vi "dfd_FXP Casting (vector).vi"(5 "quantization settings":T4={"source"=6, "wl"=1, "iwl"=1, "overflow mode"=enum."Saturation", "rounding mode"=enum."Nearest", "signed?"=TRUE} {"source" items=["Coef a/k"=0, "Coef b/v"=7, "Input"=1, "Output"=2, "Multiplicand"=3, "Product"=4, "Sum"=5, "Delay"=6, "Gain"=8]}, 6 "filtering statistics in":T3(array[cluster]) {"statistics information"."min value" format="%.2f"; "statistics information"."max value" format="%.2f"; "Quantizer Source" items=["Coefficients a/k"=0, "Coefficients b/v"=7, "Input"=1, "Output"=2, "Multiplicand"=3, "Product"=4, "Sum"=5, "Delay"=6]}, 9 "values in":dbl[](array[numeric]) format="%.2f") -> (0 "filtering statistics out":T3(array[cluster]) {"statistics information"."min value" format="%.2f"; "statistics information"."max value" format="%.2f"; "Quantizer Source" items=["Coefficients a/k"=0, "Coefficients b/v"=7, "Input"=1, "Output"=2, "Multiplicand"=3, "Product"=4, "Sum"=5, "Delay"=6]}, 2 "statistics information":T2 {"min value" format="%.2f"; "max value" format="%.2f"}, 3 "values out":dbl[](array[numeric]) format="%.2f")   [LabVIEW 2017, in "NI_DigFilter_FXP.lvlib"]
uses:
  <vilib>/addons/Digital Filter Design/NI_DigFilter_FXP.lvlib
  <vilib>/addons/Digital Filter Design/_Objects.llb/dfd_Internal Quantization Settings.ctl
  <vilib>/addons/Digital Filter Design/_Objects.llb/dfd_Internal Quantization Srcs.ctl
  <vilib>/addons/Digital Filter Design/_Objects.llb/DFD FXP Statistics Data.ctl
  <vilib>/addons/Digital Filter Design/_Objects.llb/DFD Quantization Sources.ctl
  <vilib>/addons/Digital Filter Design/FXPLib.llb/dfd_FXP Overflow (vector).vi
  <vilib>/addons/Digital Filter Design/FXPLib.llb/dfd_FXP Quantization (vector).vi
  <vilib>/addons/Digital Filter Design/NI_DigFilterLicensed.lvlib
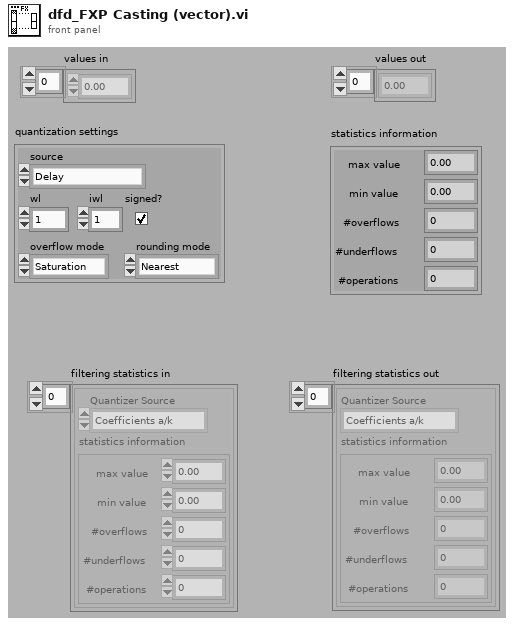
[diagram p1: front panel]
types:
  T1 = typedef "NI_DigFilterLicensed.lvlib/DFD Quantization Sources.ctl" = u16
  T2 = typedef "NI_DigFilterLicensed.lvlib/DFD FXP Statistics Data.ctl" = cluster{"max value":ext, "min value":ext, "#overflows":i32, "#underflows":i32, "#operations":i32}
  T3 = cluster{"Quantizer Source":T1, "statistics information":T2}[]
  T4 = typedef "NI_DigFilterLicensed.lvlib/dfd_Internal Quantization Settings.ctl" = cluster{"source":T5, "wl":i16, "iwl":i16, "overflow mode":enum16{"Saturation", "Wrap"}, "rounding mode":enum16{"Nearest", "Truncation"}, "signed?":bool}
  T5 = typedef "NI_DigFilterLicensed.lvlib/dfd_Internal Quantization Srcs.ctl" = u16
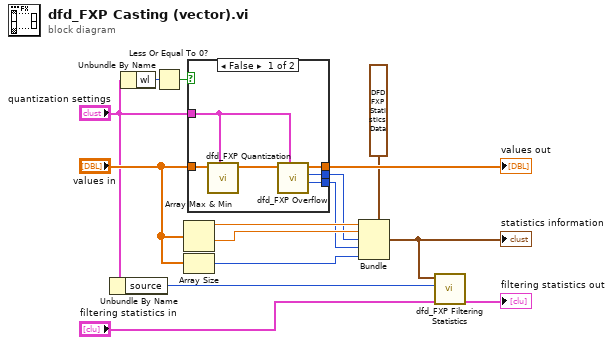
[diagram p0: block diagram]
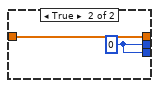
[diagram p2: hidden frame]
diagram:
  n1 = Unbundle By Name("quantization settings") -> ("source"=w3:T5)
  n2 = Unbundle By Name("quantization settings") -> ("wl"=w6:i16)
  n3 = Less Or Equal To 0?(x=w6) -> (x <= 0?=w5:bool)
  n4 = Array Max & Min(array="values in") -> (max value=w12:dbl, min value=w11:dbl)  [unwired: 2 out]
  n5 = Array Size(array="values in") -> (size(s)=w8:i32)
  n6 = case shown="False" w5 {
    tunnel: "quantization settings" -> [w20 _]
    tunnel: [w19 w23] -> w15
    tunnel: "values in" -> [w18 w23]
    tunnel: [w17 w22] -> w10
    tunnel: [w16 w22] -> w9
    frame False {
      n7 = call-poly <vilib>:"dfd_FXP Quantization.vi"("quantization settings"=w20, "values in"=w18) -> ("values out"=w21:dbl[])  [unwired: 6 out]
      n8 = call-poly <vilib>:"dfd_FXP Overflow.vi"("quantization settings"=w20, "values in"=w21) -> ("# underflow"=w16:i32, "# overflow"=w17:i32, "values out"=w19:dbl[])  [unwired: 4 out]
    }
    frame True {
      w22 = 0 ("#overflow")
    }
  }
  "values out" <- w15
  n9 = Bundle(cluster=T2 {"max value"=0.0, "min value"=0.0, "#overflows"=0, "#underflows"=0, "#operations"=0} ("statistics information"), "max value"=w12, "min value"=w11, "#overflows"=w10, "#underflows"=w9, "#operations"=w8) -> (w7:T2)
  "statistics information" <- w7
  n10 = call <vilib>:"dfd_FXP Filtering Statistics.vi"("filtering statistics in"="filtering statistics in", "source"=w3, "new data"=w7) -> ("filtering statistics out"=→"filtering statistics out":T3)  [unwired: 1 in, 7 out]
